vi "APC_9056_WatchDog.vi"() -> ()   [LabVIEW 2020]
uses:
  controls/APC_ControlSettings.ctl
  controls/APC_PIDcontrolSettings.ctl
panel:
  out "MTRnotResponding":bool
  in  "MTRwatchdogThreshold":i32
  out "PCnotResponding":bool
  in  "PCwatchdogThreshold":i32
  out "9049notResponding":bool
  in  "9049watchdogThreshold":i32
  out "9056notResponding":bool
  in  "9056watchdogThreshold":i32
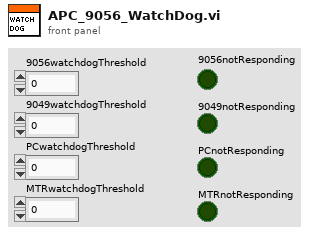
[diagram p1: front panel]
types:
  T1 = typedef "APC_ControlSettings.ctl" = cluster{"Spark advance [CADBTDC]":dbl, "Pref":dbl, "O2ref":dbl, "DI advance [CADBTDC]":dbl, "DI duration [ms] ":dbl, "CO2ref":dbl, "PFI duration [ms]":dbl, "IMEP ref":dbl, "Speed ref":dbl, "IGN enable":bool, "DI enable":bool, "CL PFI\n lambda":bool, "CL PFI\nIMEP":bool, "Activate\ncylinder":bool[], "Force idling":bool, "Force motoring":bool, "ETP resync":bool, "Requested mode":i8, "Clear Sync Errors":bool, "toggle TDC":bool, "l ref":dbl, "PID control references":T2, "CA50setpoint [CADATDC]":dbl, "CA50 control":bool, "Knock control":bool, "CLEAR EMERGENCY STOP":bool, "EMERGENCY STOP":bool}
  T2 = typedef "APC_PIDcontrolSettings.ctl" = cluster{"NG":bool, "Ar":bool, "O2":bool, "Intake vent":bool, "Cross vent":bool, "Exhaust vent":bool, "NG control mode":u8, "NG-FC-001-REF":dbl, "WF-OA-002-REF":dbl, "IMEP-REF":dbl, "Nm-REF":dbl, "Ar control mode":u8, "AR-PC-002-REF":dbl, "WF-PT-004-REF":dbl, "O2 control mode":u8, "O2-FC-001-REF":dbl, "WF-OA-001-REF":dbl, "Tcoolant control  mode":u8, "EC-FC-001-REF":dbl, "EC-TT-001-REF":dbl, "Texh control mode":u8, "SW-FC-004-REF":dbl, "SW-FT-002-REF":dbl, "WF-TT-004-REF":dbl, "Toil control mode":u8, "SW-FC-009-REF":dbl, "SW-FT-004-REF":dbl, "EO-TT-001-REF":dbl, "AIC201_CO2_ConcTarget":dbl, "O2_FF_NG":bool, "Dyno control mode":u8, "Membrane control mode":u8, "AR-FT-001-REF":dbl, "MTR modbus floats":sgl[], "MTR modbus u16":u16[], "MTR HB":bool, "PC_HB":bool, "EMERGENCY STOP":bool}
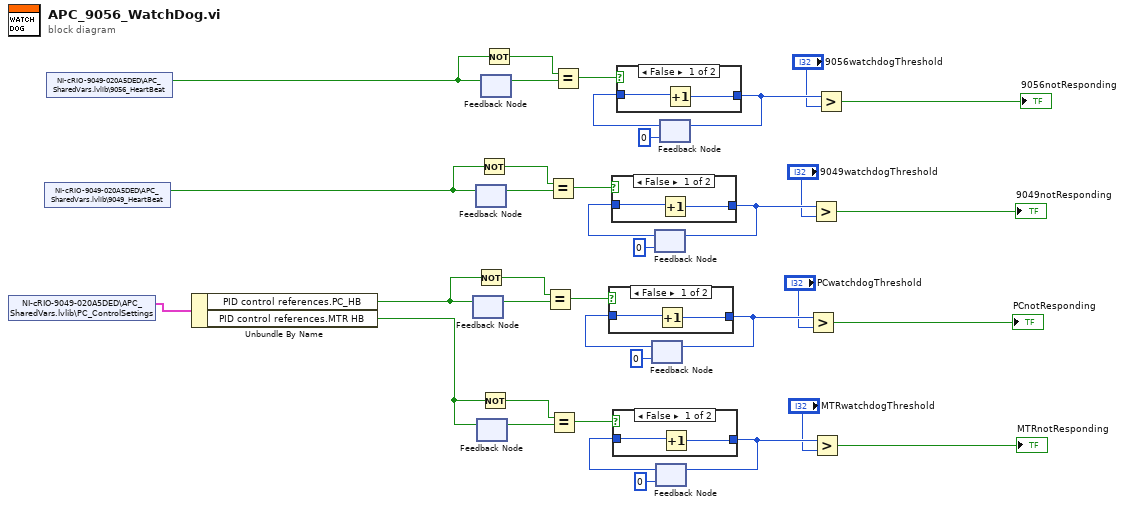
[diagram p0: block diagram]
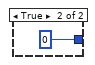
[diagram p2: hidden frame]
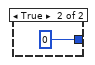
[diagram p3: hidden frame]
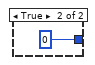
[diagram p4: hidden frame]
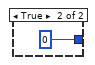
[diagram p5: hidden frame]
diagram:
  n1 = shared-variable "NI-cRIO-9049-020A5DED\\APC_SharedVars.lvlib\\PC_ControlSettings"() -> (w1:T1)  [unwired: 1 in, 1 out]
  n2 = shared-variable "NI-cRIO-9049-020A5DED\\APC_SharedVars.lvlib\\9049_HeartBeat"() -> (w20:bool)  [unwired: 1 in, 1 out]
  n3 = shared-variable "NI-cRIO-9049-020A5DED\\APC_SharedVars.lvlib\\9056_HeartBeat"() -> (w37:bool)  [unwired: 1 in, 1 out]
  n4 = Unbundle By Name(w1) -> ("PID control references.PC_HB"=w11:bool, "PID control references.MTR HB"=w2:bool)
  n5 = feedback #1() -> (w18:bool)  [unwired: 1 in]
  n6 = feedback-in #1(w11) -> ()
  n7 = feedback #2() -> (w27:bool)  [unwired: 1 in]
  n8 = feedback-in #2(w20) -> ()
  n9 = Not(x=w11) -> (.not. x?=w19:bool)
  n10 = feedback #3() -> (w9:bool)  [unwired: 1 in]
  n11 = feedback-in #3(w2) -> ()
  n12 = Not(x=w20) -> (.not. x?=w28:bool)
  n13 = Not(x=w2) -> (.not. x?=w10:bool)
  n14 = feedback-in #4(w37) -> ()
  n15 = feedback #4() -> (w35:bool)  [unwired: 1 in]
  n16 = Not(x=w37) -> (.not. x?=w36:bool)
  n17 = Equal?(x=w19, y=w18) -> (x = y?=w17:bool)
  n18 = Equal?(x=w28, y=w27) -> (x = y?=w26:bool)
  n19 = Equal?(x=w10, y=w9) -> (x = y?=w8:bool)
  n20 = Equal?(x=w36, y=w35) -> (x = y?=w34:bool)
  n21 = feedback #5(0) -> (w16:i32)
  n22 = case shown="False" w17 {
    tunnel: [w38 0] -> w14
    tunnel: w16 -> [w39 _]
    frame False {
      n23 = Increment(x=w39) -> (x+1=w38:i32)
    }
    frame True {
    }
  }
  n24 = feedback-in #5(w14) -> ()
  n25 = feedback #6(0) -> (w25:i32)
  n26 = case shown="False" w26 {
    tunnel: [w41 0] -> w23
    tunnel: w25 -> [w42 _]
    frame False {
      n27 = Increment(x=w42) -> (x+1=w41:i32)
    }
    frame True {
    }
  }
  n28 = feedback-in #6(w23) -> ()
  n29 = feedback #7(0) -> (w7:i32)
  n30 = case shown="False" w8 {
    tunnel: [w44 0] -> w5
    tunnel: w7 -> [w45 _]
    frame False {
      n31 = Increment(x=w45) -> (x+1=w44:i32)
    }
    frame True {
    }
  }
  n32 = feedback-in #7(w5) -> ()
  n33 = feedback #8(0) -> (w33:i32)
  n34 = case shown="False" w34 {
    tunnel: [w47 0] -> w31
    tunnel: w33 -> [w48 _]
    frame False {
      n35 = Increment(x=w48) -> (x+1=w47:i32)
    }
    frame True {
    }
  }
  n36 = feedback-in #8(w31) -> ()
  n37 = Greater?(x=w14, y="PCwatchdogThreshold") -> (0:→"PCnotResponding":bool)
  n38 = Greater?(x=w23, y="9049watchdogThreshold") -> (0:→"9049notResponding":bool)
  n39 = Greater?(x=w5, y="MTRwatchdogThreshold") -> (0:→"MTRnotResponding":bool)
  n40 = Greater?(x=w31, y="9056watchdogThreshold") -> (0:→"9056notResponding":bool)
